vi "Global.vi"() -> ()   [LabVIEW 2013]
panel:
  in  "SetMasterID":i32
  in  "Lap Counter":i32
  out "IsOvertaking":bool
  out "Positioned":bool
  in  "Transition WP":i32[][](array[numeric])=[[-1, -1, -1, -1], [-1, -1, -1, -1], [-1, -1, 2, 1], [-1, -1, 13, 8]]
  out "FirstTime":bool
  in  "TL  Inner":bool
  in  "TL Outer":bool
  out "ScenarioArray":u32[](array[numeric])
  in  "MasterID":i32
  in  "RealSpeed":dbl[](array[numeric])
  in  "stop":bool
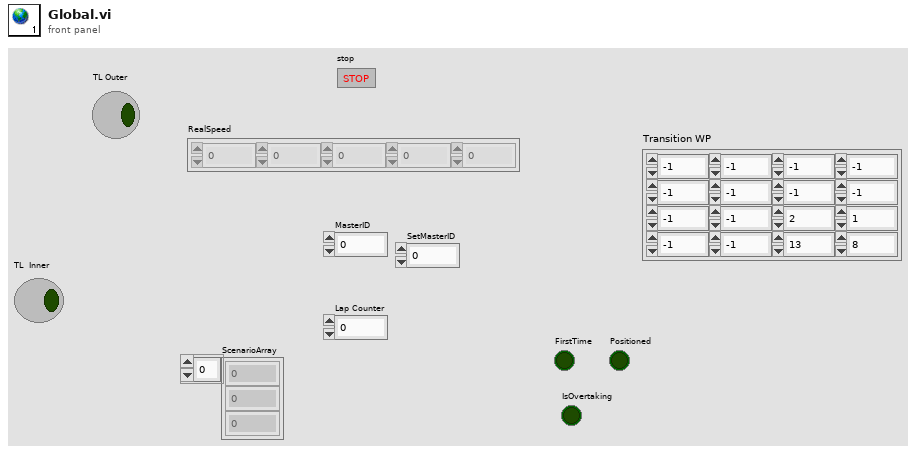
[diagram p1: front panel]
diagram:
